vi "Write Config Unitest.vi"(8 "error in (no error)":errorcluster, 11 "main ref":T1) -> (0 "error out":errorcluster)   [LabVIEW 2025]
uses:
  controls/LAB-IQ UI Data.ctl
  Traction Loop/Traction Receipe Enum.ctl
  Config file  FGV Unitest enum.ctl
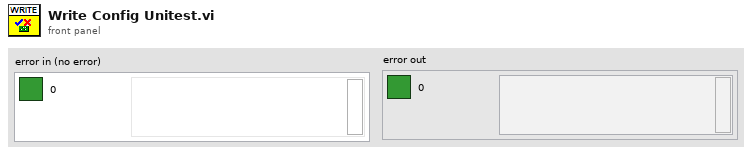
[diagram p1: front panel]
types:
  T1 = typedef "LAB-IQ UI Data.ctl" = cluster{"Main Home Screen":cluster{"GUI":refnum<vi>, "Platform Settings":refnum<vi>, "Configure":refnum<vi>, "Home":refnum<vi>, "EXIT":refnum<vi>, "service 2":refnum<vi>, "MainPage":refnum<vi>, "Analysis":refnum<vi>}, "Platform Settings":cluster{"mm/s  Surge":refnum<vi>, "Update Surge Speed":refnum<vi>, "Drive Error":refnum<vi>, "Disable Axis Jog Soft Limits":refnum<vi>, "mm/s  Sway":refnum<vi>, "Sway and Surge COM Status":refnum<vi>, "Heave COM Status":refnum<vi>, "Enable Platform":refnum<vi>, "Surge Forward Main":refnum<vi>, "Sway Right Main":refnum<vi>, "Sway Left Main":refnum<vi>, "Heave Down Main":refnum<vi>, "Heave Up main":refnum<vi>, "Update Sway Speed":refnum<vi>, "Update Heave Speed":refnum<vi>, "mm/s Heave":refnum<vi>, "mm/sec":refnum<vi>, "mm":refnum<vi>, "Surge Backward Main":refnum<vi>}, "Analysis Screen":cluster{"Analysis Home":refnum<vi>, "Surface Analysis":refnum<vi>, "Imaging":refnum<vi>, "Image Analysis":refnum<vi>, "Post Analysis":refnum<vi>}, "Config Screen":cluster{"Select Load Head":refnum<vi>, "Notes :":refnum<vi>, "FILE":refnum<vi>, "Sample ID :":refnum<vi>, "Operator ID :":refnum<vi>, "Operator Name :":refnum<vi>, "Auto":refnum<vi>}, "Motion Module":cluster{"zNL":refnum<vi>, "NL disp":refnum<vi>, "Rotary Tab":refnum<vi>, "Motion Direction:  3":refnum<vi>, "E.Velocity 2":refnum<vi>, "e.v/ssr 2":refnum<vi>, "Enter Fixed E.Velocity 2":refnum<vi>, "Enter Final SRR 2":refnum<vi>, "Enter initial SRR 2":refnum<vi>, "Enter Fixed SRR 2":refnum<vi>, "Enter the Final E.Velocity (m/s) 2":refnum<vi>, "Enter initial E.Velocity (m/s) 2":refnum<vi>, "Final Speed (RPM) 3":refnum<vi>, "Initial Speed (RPM) 2":refnum<vi>, "Enter the Final Velocity (m/s) 3":refnum<vi>, "Enter initial Velocity (m/s)  3":refnum<vi>, "Ramp Up 2":refnum<vi>, "TEST SELECTION":refnum<vi>, "SPEED SELECTION : ":refnum<vi>, "Angular Oscillation Set":refnum<vi>, "Traction":refnum<vi>, "Step Speed":refnum<vi>, "StepTable For Load-Speed":refnum<vi>, "StepTable For Speed":refnum<vi>, "Surge Forward MM":refnum<vi>, "Surge Backward MM":refnum<vi>, "M3 Image":refnum<vi>, "String 39":refnum<vi>, "Sway Left MM":refnum<vi>, "Sway Right MM":refnum<vi>, "Disable Axis Jog Soft Limits":refnum<vi>, "mm":refnum<vi>, "Heave Down MM":refnum<vi>, "Heave Up MM":refnum<vi>, "Wear Track Diameter (mm)":refnum<vi>, "Set WTD":refnum<vi>, "HomeScratch":refnum<vi>, "HomeRot":refnum<vi>, "PlaceModule":refnum<vi>, "Enter the Angle (Deg)":refnum<vi>, "Enter the Frequency (Hz)":refnum<vi>, "Motion Mode:":refnum<vi>, "LR Sway":refnum<vi>, "Rot Hor":refnum<vi>, "Scratch":refnum<vi>, "LR Cam":refnum<vi>, "MMBack":refnum<vi>, "MMNext":refnum<vi>, "Rot Ver":refnum<vi>, "Rotary Module Selection":refnum<vi>, "calculate rotary":refnum<vi>, "SPEED SELECTION : rotary":refnum<vi>, "Import 2":refnum<vi>, "Save 2":refnum<vi>, "File Path :  2":refnum<vi>, "String 45":refnum<vi>, "StepTable For Speed 3":refnum<vi>, "Enter the Speed(mm/sec)":refnum<vi>, "Enter the Speed(RPM)":refnum<vi>, "Enter Scratch Speed (mm/s):":refnum<vi>, "SwaySpeed Set":refnum<vi>, "Scartch Offset":refnum<vi>, "Motion type:":refnum<vi>, "HomeScratch 2":refnum<vi>, "Enter Scratch length (mm):":refnum<vi>, "Wear Track Diameter":refnum<vi>, "Rotary Speed Exced":refnum<vi>, "Scratch Mode":refnum<vi>, "No of Scratch":refnum<vi>}, "Environmental control":cluster{"Humidity  Status  3":refnum<vi>, "Low Temp  Status  2":refnum<vi>, "TK4 status 2":refnum<vi>, "Stage Temperature":refnum<vi>, "Sample Temperature":refnum<vi>, "Humidity (Amb)":refnum<vi>, "Clear List":refnum<vi>, "Add to list":refnum<vi>, "Wear":refnum<vi>, "Vibration":refnum<vi>, "Humidity (Chamber)":refnum<vi>, "Temperature (Chamber)":refnum<vi>, "ECR ":refnum<vi>, "Temperature (Amb)":refnum<vi>, "Microphone":refnum<vi>, "Acoustic Emission 3":refnum<vi>, "SNext":refnum<vi>, "APBack":refnum<vi>, "Enter the Temperature (°C):":refnum<vi>, "Enter the Stage \nTemperature (°C):":refnum<vi>, "Enter the Humidity (%Rh):":refnum<vi>, "Low Temp":refnum<vi>, "High Temp":refnum<vi>, "Humidity":refnum<vi>, "Sensors Picked":refnum<vi>}, "About Screen":cluster{"Password":refnum<vi>, "Home Service":refnum<vi>, "Advanced Setting":refnum<vi>, "About Tab":refnum<vi>, "ECR Port:":refnum<vi>, "Ramp Port:":refnum<vi>, "Installation/Replacement completed":refnum<vi>, "Loahead":refnum<vi>, "Heave and Surge COM Port:":refnum<vi>, "Sway COM Port:":refnum<vi>, "Temp Modbus:":refnum<vi>, "Humidity Port:":refnum<vi>, "Edit Gain Constants":refnum<vi>, "Save Gain Constants":refnum<vi>}, "Main Screen":cluster{"Main Screen Tab":refnum<vi>, "Angle and Frequency":refnum<vi>, "Stroke (mm)":refnum<vi>, "Angle (Deg)":refnum<vi>, "Main Speed Tab":refnum<vi>, "MTM MOTOR DISPLAY":refnum<vi>, "Disc Speed (m/sec)":refnum<vi>, "Ball Speed (m/sec)":refnum<vi>, "Disc Speed (RPM)":refnum<vi>, "Ball Speed (RPM)":refnum<vi>, "SPEED TAB":refnum<vi>, "Speed (m/sec)":refnum<vi>, "Set Speed (m/sec)":refnum<vi>, "Speed (RPM)":refnum<vi>, "Set Speed":refnum<vi>, "Time Tab":refnum<vi>, "Time ( HH:MM:SS ) 2":refnum<vi>, "Test Duration":refnum<vi>, "Test Duration 4":refnum<vi>, "TEST CYCLE":refnum<vi>, "TOTAL CYCLES":refnum<vi>, "Set Load (N)":refnum<vi>, "Temp Tabs":refnum<vi>, "Heater":refnum<vi>, "TK4 status":refnum<vi>, "ChamberTemp":refnum<vi>, "SetTmp":refnum<vi>, "Controller  Status":refnum<vi>, "ChamberTemp 2":refnum<vi>, "SetTmp 2":refnum<vi>, "Controller  Status 2":refnum<vi>, "ChamberTemp 3":refnum<vi>, "SetTmp 3":refnum<vi>, "Cooling":refnum<vi>, "Load Communication":refnum<vi>, "Ambient \nTemperature":refnum<vi>, "HumCOMStatus":refnum<vi>, "Ambient\n Humidity":refnum<vi>, "Freq (Hz)":refnum<vi>, "Load En":refnum<vi>, "NLt":refnum<vi>, "zNL 2":refnum<vi>, "Humidity On":refnum<vi>, "humidity disp":refnum<vi>, "Set Humidity":refnum<vi>, "NL disp 2":refnum<vi>, "Humidity On 2":refnum<vi>, "humidity disp 2":refnum<vi>, "Set Humidity 2":refnum<vi>, "NL disp 3":refnum<vi>, "AppLoadSeq scratch":refnum<vi>, "Stop Scratch":refnum<vi>, "ClrLog":refnum<vi>, "Trip Log":refnum<vi>, "STOP":refnum<vi>, "Start Test":refnum<vi>, "Test status":refnum<vi>, "AR Led":refnum<vi>, "Data":refnum<vi>, "Health":refnum<vi>, "Sway COM Status":refnum<vi>, "Heave COM Status":refnum<vi>, "Grp Tab":refnum<vi>, "Sub Graph":refnum<vi>, "SD (mm)":refnum<vi>, "Siliding distance Reset Graph":refnum<vi>, "SDGp":refnum<vi>, "Humidity Reset Graph":refnum<vi>, "HumrGp":refnum<vi>, "Acoustic Emission (mV)":refnum<vi>, "Aqucostic Reset Graph":refnum<vi>, "gACQUOS":refnum<vi>, "ECR RESET":refnum<vi>, "ECR":refnum<vi>, "Temperature Reset":refnum<vi>, "Acoustic Emission (mV) 2":refnum<vi>, "Aqucostic Reset Graph 2":refnum<vi>, "gACQUOS 2":refnum<vi>, "ECR RESET 2":refnum<vi>, "ECR 2":refnum<vi>, "Temperature Reset 2":refnum<vi>, "Temperature (deg c)":refnum<vi>, "Speed Reset Graph":refnum<vi>, "Speed Tab":refnum<vi>, "MTM DISC  SPEED":refnum<vi>, "MTM BALL SPEED":refnum<vi>, "speed mm/sec":refnum<vi>, "Hymidity":refnum<vi>, "Humidity Disable trip":refnum<vi>, "CoF Trip  2":refnum<vi>, "Depth Trip":refnum<vi>, "Weart Deapth":refnum<vi>, "Depth Reset Graph":refnum<vi>, "Weart":refnum<vi>, "Depthz":refnum<vi>, "Depth (µm)":refnum<vi>, "WearGp":refnum<vi>, "NL Trip 2":refnum<vi>, "Load pid":refnum<vi>, "Load Disable Trip":refnum<vi>, "Load Reset Graph":refnum<vi>, "NL Display 4":refnum<vi>, "Main Chart 3":refnum<vi>, "BACK":refnum<vi>, "Depth Trip 2":refnum<vi>, "COF TRIP ":refnum<vi>, "Friction Force (N)":refnum<vi>, "FF Reset Graph":refnum<vi>, "FF Disable Trip":refnum<vi>, "FF TRIP":refnum<vi>, "COF Disable Trip":refnum<vi>, "COF Reset Graph":refnum<vi>, "Start Test Temp":refnum<vi>, "zFF":refnum<vi>, "Friction Force (N) Graph":refnum<vi>, "Coefficient of Friction":refnum<vi>, "Scratch Start Test":refnum<vi>, "FF Tab":refnum<vi>, "Cyclic Friction Force (N)":refnum<vi>, "CZ FF":refnum<vi>, "Cyclic Friction Force (N) Graph":refnum<vi>, "Cyclic Coefficient of Friction":refnum<vi>, "Cyclic FF TRIP":refnum<vi>, "Cyclic FF Disable Trip":refnum<vi>, "cyclic COF Disable Trip":refnum<vi>, "cyclic COF TRIP":refnum<vi>, "cyclic COF Reset Graph":refnum<vi>, "Cyclic FF Reset Graph":refnum<vi>, "Test Trip":refnum<vi>, "Multi Scratch Pass":refnum<vi>, "Scratch Start Recording":refnum<vi>}, "Loading":cluster{"Indentation":refnum<vi>, "Reference Sample":refnum<vi>, "Load Cell Communication Slide":refnum<vi>, "com 3":refnum<vi>, "com":refnum<vi>, "DecaForce COM Status":refnum<vi>, "Update":refnum<vi>, "Clear 3":refnum<vi>, "seq":refnum<vi>, "Stribeck table":refnum<vi>, "Stribeck Table  For loading":refnum<vi>, "Loading Mode":refnum<vi>, "Enter the Final Load (N)":refnum<vi>, "Enter the CoF Trip":refnum<vi>, "Enter the Friction Force Trip":refnum<vi>, "Enter the Normal load Trip":refnum<vi>, "Enter the Load  (N)":refnum<vi>, "KiloForce":refnum<vi>, "DecaForce ":refnum<vi>, "MicroForce":refnum<vi>, "LHBack":refnum<vi>, "LHNext":refnum<vi>, "Enter the Loading Rate (N/min)":refnum<vi>, "Message":refnum<vi>, "Warning 2":refnum<vi>, "SSP 0.75":refnum<vi>, "SSP 0.5":refnum<vi>, "SSP 0.3":refnum<vi>, "Warning":refnum<vi>, "gui GIF":refnum<vi>, "Communication is established":refnum<vi>, "AppLoad 4":refnum<vi>, "Multipoint":refnum<vi>, "Load Selection":refnum<vi>}, "PID":cluster{"Ramp MulFac":refnum<vi>, "pulses LoadDiffRamp(2..10)":refnum<vi>, "PulseControlRamp(diff<=3N)":refnum<vi>, "SetLoadDeadband(%) Load(0-10N)":refnum<vi>, "PID gains out delay (microForce)":refnum<vi>, "Ramp":refnum<vi>, "Gain 2":refnum<vi>, "pulses LoadDiff(2..10)":refnum<vi>, "pulses LoadDiff(11..50)":refnum<vi>, "PulseControl(diff<=3N)":refnum<vi>, "SetLoadDeadband(%)  2":refnum<vi>, "Dummy Run":refnum<vi>, "Vertical load (N)":refnum<vi>, "AutoTune":refnum<vi>, "Offset 3 ":refnum<vi>, "apply load":refnum<vi>, "Offset  3":refnum<vi>, "apply load 2":refnum<vi>, "Enter ByPass Load":refnum<vi>, "reinit 3":refnum<vi>, "output range delay":refnum<vi>, "PID gains out delay":refnum<vi>, "Bypass Load":refnum<vi>, "pulsesSent":refnum<vi>, "pulses ":refnum<vi>, "actpid":refnum<vi>, "gFF Rot":refnum<vi>, "pulses LoadDiff(21..1000)":refnum<vi>, "Delay":refnum<vi>, "deadband":refnum<vi>}, "Config Parameters":cluster{"Tab Control 3":refnum<vi>, "Tab Control 19":refnum<vi>, "SAMPLES":refnum<vi>, "Re-initilaize":refnum<vi>, "Filter ON/OFF":refnum<vi>, "TracHomeSurgeOffsetCounts 10MM":refnum<vi>, "TracHomeSwayOffsetCounts 10MM":refnum<vi>, "Acoustic Emission:":refnum<vi>, "Apply Filter (FF)":refnum<vi>, "Filter% 2":refnum<vi>, "Apply Filter (Load)":refnum<vi>, "Filter% ":refnum<vi>, "Sway distance (mm)":refnum<vi>, "Surge distance (mm)":refnum<vi>, "DataSavingLoopDelay(ms)":refnum<vi>, "SAVE 2":refnum<vi>, "Enter Distance":refnum<vi>, "Sway Counts:":refnum<vi>, "Distance (mm): 3":refnum<vi>, "Surge Counts:":refnum<vi>, "Distance (mm): 2":refnum<vi>, "Distance (mm):":refnum<vi>, "Heave Counts:":refnum<vi>, "LRMHomeSurgeOffsetCounts":refnum<vi>, "LRMHomeSwayOffsetCounts":refnum<vi>, "TracHomeSurgeOffsetCounts 20MM":refnum<vi>, "TracHomeSwayOffsetCounts 20MM":refnum<vi>, "RotHomeSwayOffsetCounts":refnum<vi>, "RotHomeSurgeOffsetCounts":refnum<vi>, "Heave distance":refnum<vi>, "Zmm":refnum<vi>, "Heave Pulses/mm":refnum<vi>, "Surge Pulses/mm":refnum<vi>, "Sway Pulses/mm":refnum<vi>, "Heave Pitch":refnum<vi>, "Surge Pitch":refnum<vi>, "Sway Pitch":refnum<vi>, "Heave PPR":refnum<vi>, "Surge PPR":refnum<vi>, "Sway PPR":refnum<vi>, "Tab Control 5":refnum<vi>, "Tab Control 14":refnum<vi>, "Tab Control 26":refnum<vi>, "AE":refnum<vi>, "Heave Loop Delay":refnum<vi>, "Heave PID Speed":refnum<vi>, "Surge Jog Speed":refnum<vi>, "Heave Jog Speed":refnum<vi>, "Sway Loop Delay":refnum<vi>, "Sway PID Speed":refnum<vi>, "Sway Jog Speed":refnum<vi>, "DEPTH TRIP VALUE":refnum<vi>, "LOAD TRIP VALUE":refnum<vi>, "DEPTH TRIP   ENABLE":refnum<vi>, "LOAD TRIP  ENABLE":refnum<vi>, "CYCLIC FF TRIP VALUE":refnum<vi>, "FF TRIP VALUE":refnum<vi>, "CYCLIC CoF TRIP VALUE":refnum<vi>, "COF TRIP VALUE":refnum<vi>, "CYCLIC COF TRIP  ENABLE":refnum<vi>, "CYCLIC FF TRIP  ENABLE":refnum<vi>, "FF TRIP  ENABLE":refnum<vi>, "COF TRIP  ENABLE":refnum<vi>, "JOG TRIP LOAD VALUE (N)":refnum<vi>, "Rotary Vertical":refnum<vi>, "Traction":refnum<vi>, "Scratch":refnum<vi>, "LRM CAM":refnum<vi>, "Sway LRM":refnum<vi>, "Rotary Horizontal":refnum<vi>}, "Loading Com Port":cluster{"ClearAll":refnum<vi>, "Mz(Nm)":refnum<vi>, "My(Nm)":refnum<vi>, "Mx(Nm)":refnum<vi>, "Save Dwell":refnum<vi>, "Mx ":refnum<vi>, "My ":refnum<vi>, "Mz":refnum<vi>, "Fx(N)":refnum<vi>, "Fy(N)":refnum<vi>, "Fz(N)":refnum<vi>, "ZeroAll":refnum<vi>, "Acq Delay (ms)":refnum<vi>, "Burst Delay (ms)":refnum<vi>, "model":refnum<vi>, "SN":refnum<vi>, "FFx(N)":refnum<vi>, "Sensor IP":refnum<vi>, "Port":refnum<vi>, "FFy(N)":refnum<vi>, "Load(N)":refnum<vi>, "delete Handle":refnum<vi>, "Create Handle":refnum<vi>, "ft_data":refnum<vi>, "ft_range":refnum<vi>, "ft_data 2":refnum<vi>, "stop 6":refnum<vi>, "running_flag":refnum<vi>, "ft_udp_handle":refnum<vi>, "get-data-return":refnum<vi>, "get-range-return":refnum<vi>, "zero-return":refnum<vi>, "filter-return":refnum<vi>, "initial-return":refnum<vi>, "deleteHandle-result":refnum<vi>, "Load Cell Temp":refnum<vi>, "Load Cell":refnum<vi>}, "Heave AND Surge":cluster{"SURGE POSE":refnum<vi>, "error out Read":refnum<vi>, "HEAVE POSE":refnum<vi>, "State":refnum<vi>, "Homed":refnum<vi>, "Sequence ID":refnum<vi>, "error out Write":refnum<vi>, "faultCode":refnum<vi>, "Ack ID":refnum<vi>, "SPEED":refnum<vi>, "Distance":refnum<vi>, "Mode Command":refnum<vi>, "Heave and Surge Read":refnum<vi>, "Read Heave Temp":refnum<vi>, "Spare 15":refnum<vi>, "Spare 14":refnum<vi>, "Spare 13":refnum<vi>, "Spare 12":refnum<vi>, "Spare 11":refnum<vi>, "Spare 10":refnum<vi>, "Spare 9":refnum<vi>, "Spare 8":refnum<vi>, "Spare 7":refnum<vi>, "Spare 6":refnum<vi>, "Spare 5":refnum<vi>, "Spare 4":refnum<vi>, "Spare 2":refnum<vi>, "Spare 1":refnum<vi>, "Node Id":refnum<vi>, "Spare 3":refnum<vi>, "SPARE 4":refnum<vi>, "SPARE 3":refnum<vi>, "SPARE 2":refnum<vi>, "SPARE 1":refnum<vi>, "fwMajor":refnum<vi>, "fwMinor":refnum<vi>, "Manual Write":refnum<vi>, "Heave and Surge Write":refnum<vi>, "SPARE 5":refnum<vi>, "Reserved ":refnum<vi>, "SPARE 8":refnum<vi>, "SPARE 6":refnum<vi>, "SPARE 7":refnum<vi>, "SPARE 17":refnum<vi>, "SPARE 16":refnum<vi>, "SPARE 15":refnum<vi>, "SPARE 14":refnum<vi>, "SPARE 13":refnum<vi>, "SPARE 12":refnum<vi>, "SPARE 11":refnum<vi>, "SPARE 10":refnum<vi>, "SPARE 9":refnum<vi>, "System UPTIME":refnum<vi>, "Missed Packets":refnum<vi>, "faultCode Surge Right":refnum<vi>, "faultCode Surge Left":refnum<vi>, "faultCode Heave":refnum<vi>, "UPLINK HEAVE":refnum<vi>, "DOWNLINK HEAVE":refnum<vi>}, "New PID LOGIC":cluster{"Fine Tune Zone":refnum<vi>, "PID SDelay":refnum<vi>, "Max_pos_limit":refnum<vi>, "Min_pos_limit":refnum<vi>, "i_limit":refnum<vi>, "pct_scale":refnum<vi>, "Deadband":refnum<vi>, "Kd":refnum<vi>, "Ki":refnum<vi>, "Kp":refnum<vi>, "Current Position":refnum<vi>, "Set Load":refnum<vi>, "Current Load":refnum<vi>, "Pulse delta":refnum<vi>, "Init Step":refnum<vi>, "Max Step Linit":refnum<vi>, "min_deadband_floor":refnum<vi>, "dynamic_spindle_noise_scalar":refnum<vi>, "min_finetune_floor":refnum<vi>, "filter_alpha":refnum<vi>, "PID":refnum<vi>}, "SWAY ":cluster{"fwMajor":refnum<vi>, "Homed":refnum<vi>, "Rotary POSE":refnum<vi>, "State":refnum<vi>, "SWAY POSE":refnum<vi>, "Ack ID":refnum<vi>, "faultCode":refnum<vi>, "Node Id":refnum<vi>, "fwMinor":refnum<vi>, "Spare 6":refnum<vi>, "Spare 5":refnum<vi>, "Spare 4":refnum<vi>, "Spare 3":refnum<vi>, "Spare 2":refnum<vi>, "Spare 1":refnum<vi>, "Spare 7":refnum<vi>, "SPARE  5":refnum<vi>, "error out Write  SWAY ":refnum<vi>, "error out Read SWAY ":refnum<vi>, "Manual Write SWAY ":refnum<vi>, "SWAY WRITE":refnum<vi>, "SPARE  4":refnum<vi>, "SPARE  3":refnum<vi>, "SPARE 2":refnum<vi>, "SPARE 1":refnum<vi>, "Spare 15":refnum<vi>, "Spare 14":refnum<vi>, "Spare 13":refnum<vi>, "Spare 12":refnum<vi>, "Spare 11":refnum<vi>, "Spare 9":refnum<vi>, "Spare 8":refnum<vi>, "SPEED":refnum<vi>, "Distance":refnum<vi>, "Mode Command":refnum<vi>, "Sequence ID":refnum<vi>, "SWAY READ":refnum<vi>, "Spare 10":refnum<vi>, "Read SWAY Temp":refnum<vi>, "faultCode Sway ":refnum<vi>, "Missed Packets":refnum<vi>, "System UPTIME sway":refnum<vi>, "SPARE 6":refnum<vi>, "SPARE 7":refnum<vi>, "SPARE 9":refnum<vi>, "SPARE 11":refnum<vi>, "SPARE 10":refnum<vi>, "SPARE 8":refnum<vi>, "SPARE 13":refnum<vi>, "SPARE 12":refnum<vi>, "SPARE 17":refnum<vi>, "SPARE 16":refnum<vi>, "SPARE 15":refnum<vi>, "SPARE 14":refnum<vi>, "Reserved":refnum<vi>, "faultCode Rotary":refnum<vi>, "UPLINK SWAY":refnum<vi>, "DOWNLINK SWAY":refnum<vi>}, "Analysis Screen":cluster{"Analysis Home":refnum<vi>, "Refresh 2":refnum<vi>, "MEAN 4":refnum<vi>, "SD 4":refnum<vi>, "VARIANCE 4":refnum<vi>, "MEAN  3":refnum<vi>, "SD  3":refnum<vi>, "VARIANCE  3":refnum<vi>, "MEAN 2":refnum<vi>, "SD  2":refnum<vi>, "VARIANCE 2":refnum<vi>, "MEAN":refnum<vi>, "SD":refnum<vi>, "VARIANCE":refnum<vi>, "File 4 Discription":refnum<vi>, "OPEN 4":refnum<vi>, "File Name 4":refnum<vi>, "OPEN 3":refnum<vi>, "File 3 Discription":refnum<vi>, "File Name 3":refnum<vi>, "Y-AXIS":refnum<vi>, "X-AXIS":refnum<vi>, "XY Graph":refnum<vi>, "File Name 2":refnum<vi>, "File Name 1":refnum<vi>, "OPEN 2":refnum<vi>, "OPEN 1":refnum<vi>, "File 1 Discription ":refnum<vi>, "File 2 Discription":refnum<vi>, "Export":refnum<vi>, "File Format":refnum<vi>}, "Traction":cluster{"faultCode Traction 2":refnum<vi>, "faultCode Traction 1":refnum<vi>, "Missed Packets":refnum<vi>, "System UPTIME Traction":refnum<vi>, "SPARE 17":refnum<vi>, "SPARE 16":refnum<vi>, "SPARE 15":refnum<vi>, "SPARE 14":refnum<vi>, "SPARE 13":refnum<vi>, "SPARE 12":refnum<vi>, "SPARE 11":refnum<vi>, "SPARE 10":refnum<vi>, "SPARE 9":refnum<vi>, "SPARE 8":refnum<vi>, "SPARE 7":refnum<vi>, "SPARE 6":refnum<vi>, "Reserved":refnum<vi>, "SPARE  5":refnum<vi>, "Manual Write TRACTION":refnum<vi>, "TRACTION WRITE":refnum<vi>, "SPARE  4":refnum<vi>, "SPARE  3":refnum<vi>, "SPARE 2":refnum<vi>, "SPARE 1":refnum<vi>, "Spare 7":refnum<vi>, "Spare 6":refnum<vi>, "Spare 5":refnum<vi>, "Spare 4":refnum<vi>, "Spare 2":refnum<vi>, "Spare 1":refnum<vi>, "Node Id":refnum<vi>, "Read TRACTION Temp":refnum<vi>, "fwMinor":refnum<vi>, "fwMajor":refnum<vi>, "faultCode":refnum<vi>, "TRACTION POSE":refnum<vi>, "TRACTION POSE 2":refnum<vi>, "Homed":refnum<vi>, "State":refnum<vi>, "Ack ID":refnum<vi>, "SPEED":refnum<vi>, "Distance":refnum<vi>, "Mode Command":refnum<vi>, "Sequence ID":refnum<vi>, "error out Read TRACTION":refnum<vi>, "error out Write  TRACTION":refnum<vi>, "TRACTION READ":refnum<vi>, "Spare 3":refnum<vi>, "Downlink traction":refnum<vi>, "Uplink Traction":refnum<vi>}, "Traction reciepe":cluster{"SRR Sweep Range (%) Stribeck":refnum<vi>, "Traction Receipe":refnum<vi>, "Total Execution Time":refnum<vi>, "Total Steps":refnum<vi>, "Duration / Step (s)  Stribeck":refnum<vi>, "STRIBECK Fixed SRR List (%)":refnum<vi>, "Duration / Step (s) Traction":refnum<vi>, "SRR Sweep Range (%) traction":refnum<vi>, "Rolling Speed (mm/s)":refnum<vi>, "Temperature Stages (°C)":refnum<vi>, "Ball Load (N)":refnum<vi>, "Lubricant Name":refnum<vi>, "Profile File Name":refnum<vi>, "SET entrainment Velocity":refnum<vi>, "Test Array Size":refnum<vi>, "SRR INDEX [ STRIBECK]":refnum<vi>, "Stribeck Size":refnum<vi>, "SET SRR":refnum<vi>, "ELAPSED TIMER ":refnum<vi>, "BALL SET RPM":refnum<vi>, "DISC SET RPM":refnum<vi>, "SET LOAD":refnum<vi>, "TEMPERATURE READ":refnum<vi>, "SET TEMPERATURE":refnum<vi>, "Traction Size":refnum<vi>, "DISC SPEED (rpm)":refnum<vi>, "BALL SPEED (rpm)":refnum<vi>, "BALL WEAR TRACK":refnum<vi>, "DISC WEARTRACK":refnum<vi>, "SRR INDEX [ TRACTION]":refnum<vi>, "Start Index Type":refnum<vi>, "Enum - Menu":refnum<vi>, "Ball (mm/sec)":refnum<vi>, "Disc (mm/sec)":refnum<vi>}, "Traction Control":cluster{"HomeTraction":refnum<vi>, "Demo Mode Display":refnum<vi>, "Traction Message":refnum<vi>, "Traction Step Update Details":refnum<vi>, "Main Tab sequence for selection":refnum<vi>, "Ramp Tab":refnum<vi>, "e.v/ssr":refnum<vi>, "Enter Fixed E.Velocity":refnum<vi>, "Enter Final SRR":refnum<vi>, "Enter initial SRR":refnum<vi>, "Enter Fixed SRR":refnum<vi>, "Enter the Final E.Velocity (m/s)":refnum<vi>, "Enter initial E.Velocity (m/s)":refnum<vi>, "Ball WTD":refnum<vi>, "E.Velocity":refnum<vi>, "Enter the Final Velocity (m/s)":refnum<vi>, "Enter initial Velocity (m/s)":refnum<vi>, "Ramp Up   Disc":refnum<vi>, "Initial DiscSpeed (RPM)":refnum<vi>, "Final Speed (RPM) Ball":refnum<vi>, "Final Speed (RPM)":refnum<vi>, "Initial Speed (RPM) Ball":refnum<vi>, "Enter the Final Velocity (m/s) Ball":refnum<vi>, "Enter initial Velocity (m/s) Ball":refnum<vi>, "Ramp Up":refnum<vi>, "ExceedBallSpeed step":refnum<vi>, "ExceedDiscSpeed":refnum<vi>, "BallSpeed Exceed Indication":refnum<vi>, "Apply":refnum<vi>, "SPEED SELECTION : MTM":refnum<vi>, "SPEED SELECTION : MTM 2":refnum<vi>, "TEST SELECTION (MTM)":refnum<vi>, "MTM Test Selection":refnum<vi>, "File Path Tab":refnum<vi>, "File Path String":refnum<vi>, "Save":refnum<vi>, "Save  2":refnum<vi>, "Import ":refnum<vi>, "File Path :":refnum<vi>, "Step Sequence Indication Tab":refnum<vi>, "Step Sequence Indication":refnum<vi>, "Calculate Step":refnum<vi>, "StepTable":refnum<vi>, "ExceedDiscSpeed  Cinstant Speed":refnum<vi>, "ExceedBallSpeed Constant":refnum<vi>, "TEST SELECTION (MTM) 2":refnum<vi>, "SPEED SELECTION : MTM 3":refnum<vi>, "MTM Test Selection 2":refnum<vi>, "Enter the Speed (m/sec): ":refnum<vi>, "Enter the Speed (m/sec):  2":refnum<vi>, "Enter the Speed (RPM):":refnum<vi>, "Lower Spped ":refnum<vi>, "Upper":refnum<vi>, "Enter the Speed (RPM):Ball":refnum<vi>, "Disc Motion Direction: ":refnum<vi>, "Ball Motion Direction :":refnum<vi>, "Motion Mode: ":refnum<vi>, "Wear Track Diameter (mm) ":refnum<vi>, "Disc Speed Indicator":refnum<vi>, "ExceedBallSpeed":refnum<vi>}, "Acquostic":cluster{"Last Config Rejected ":refnum<vi>, "rx command count":refnum<vi>, "Current Filter Id":refnum<vi>, "Isolated Gain":refnum<vi>, "DAQ Status":refnum<vi>, "error out":refnum<vi>, "error in (no error)":refnum<vi>, "Uplink Packet":refnum<vi>, "data out":refnum<vi>, "Downlink Packet":refnum<vi>, "Signal Energy":refnum<vi>, "Amplitude db_AE":refnum<vi>, "Peak Amplitude":refnum<vi>, "AE Ring-Down Counts":refnum<vi>, "Gains":refnum<vi>, "Manual Write Acquostic":refnum<vi>}}
  T2 = typedef "Config file  FGV Unitest enum.ctl" = enum16{"OPEN", "READ", "WRITE", "CLOSE"}
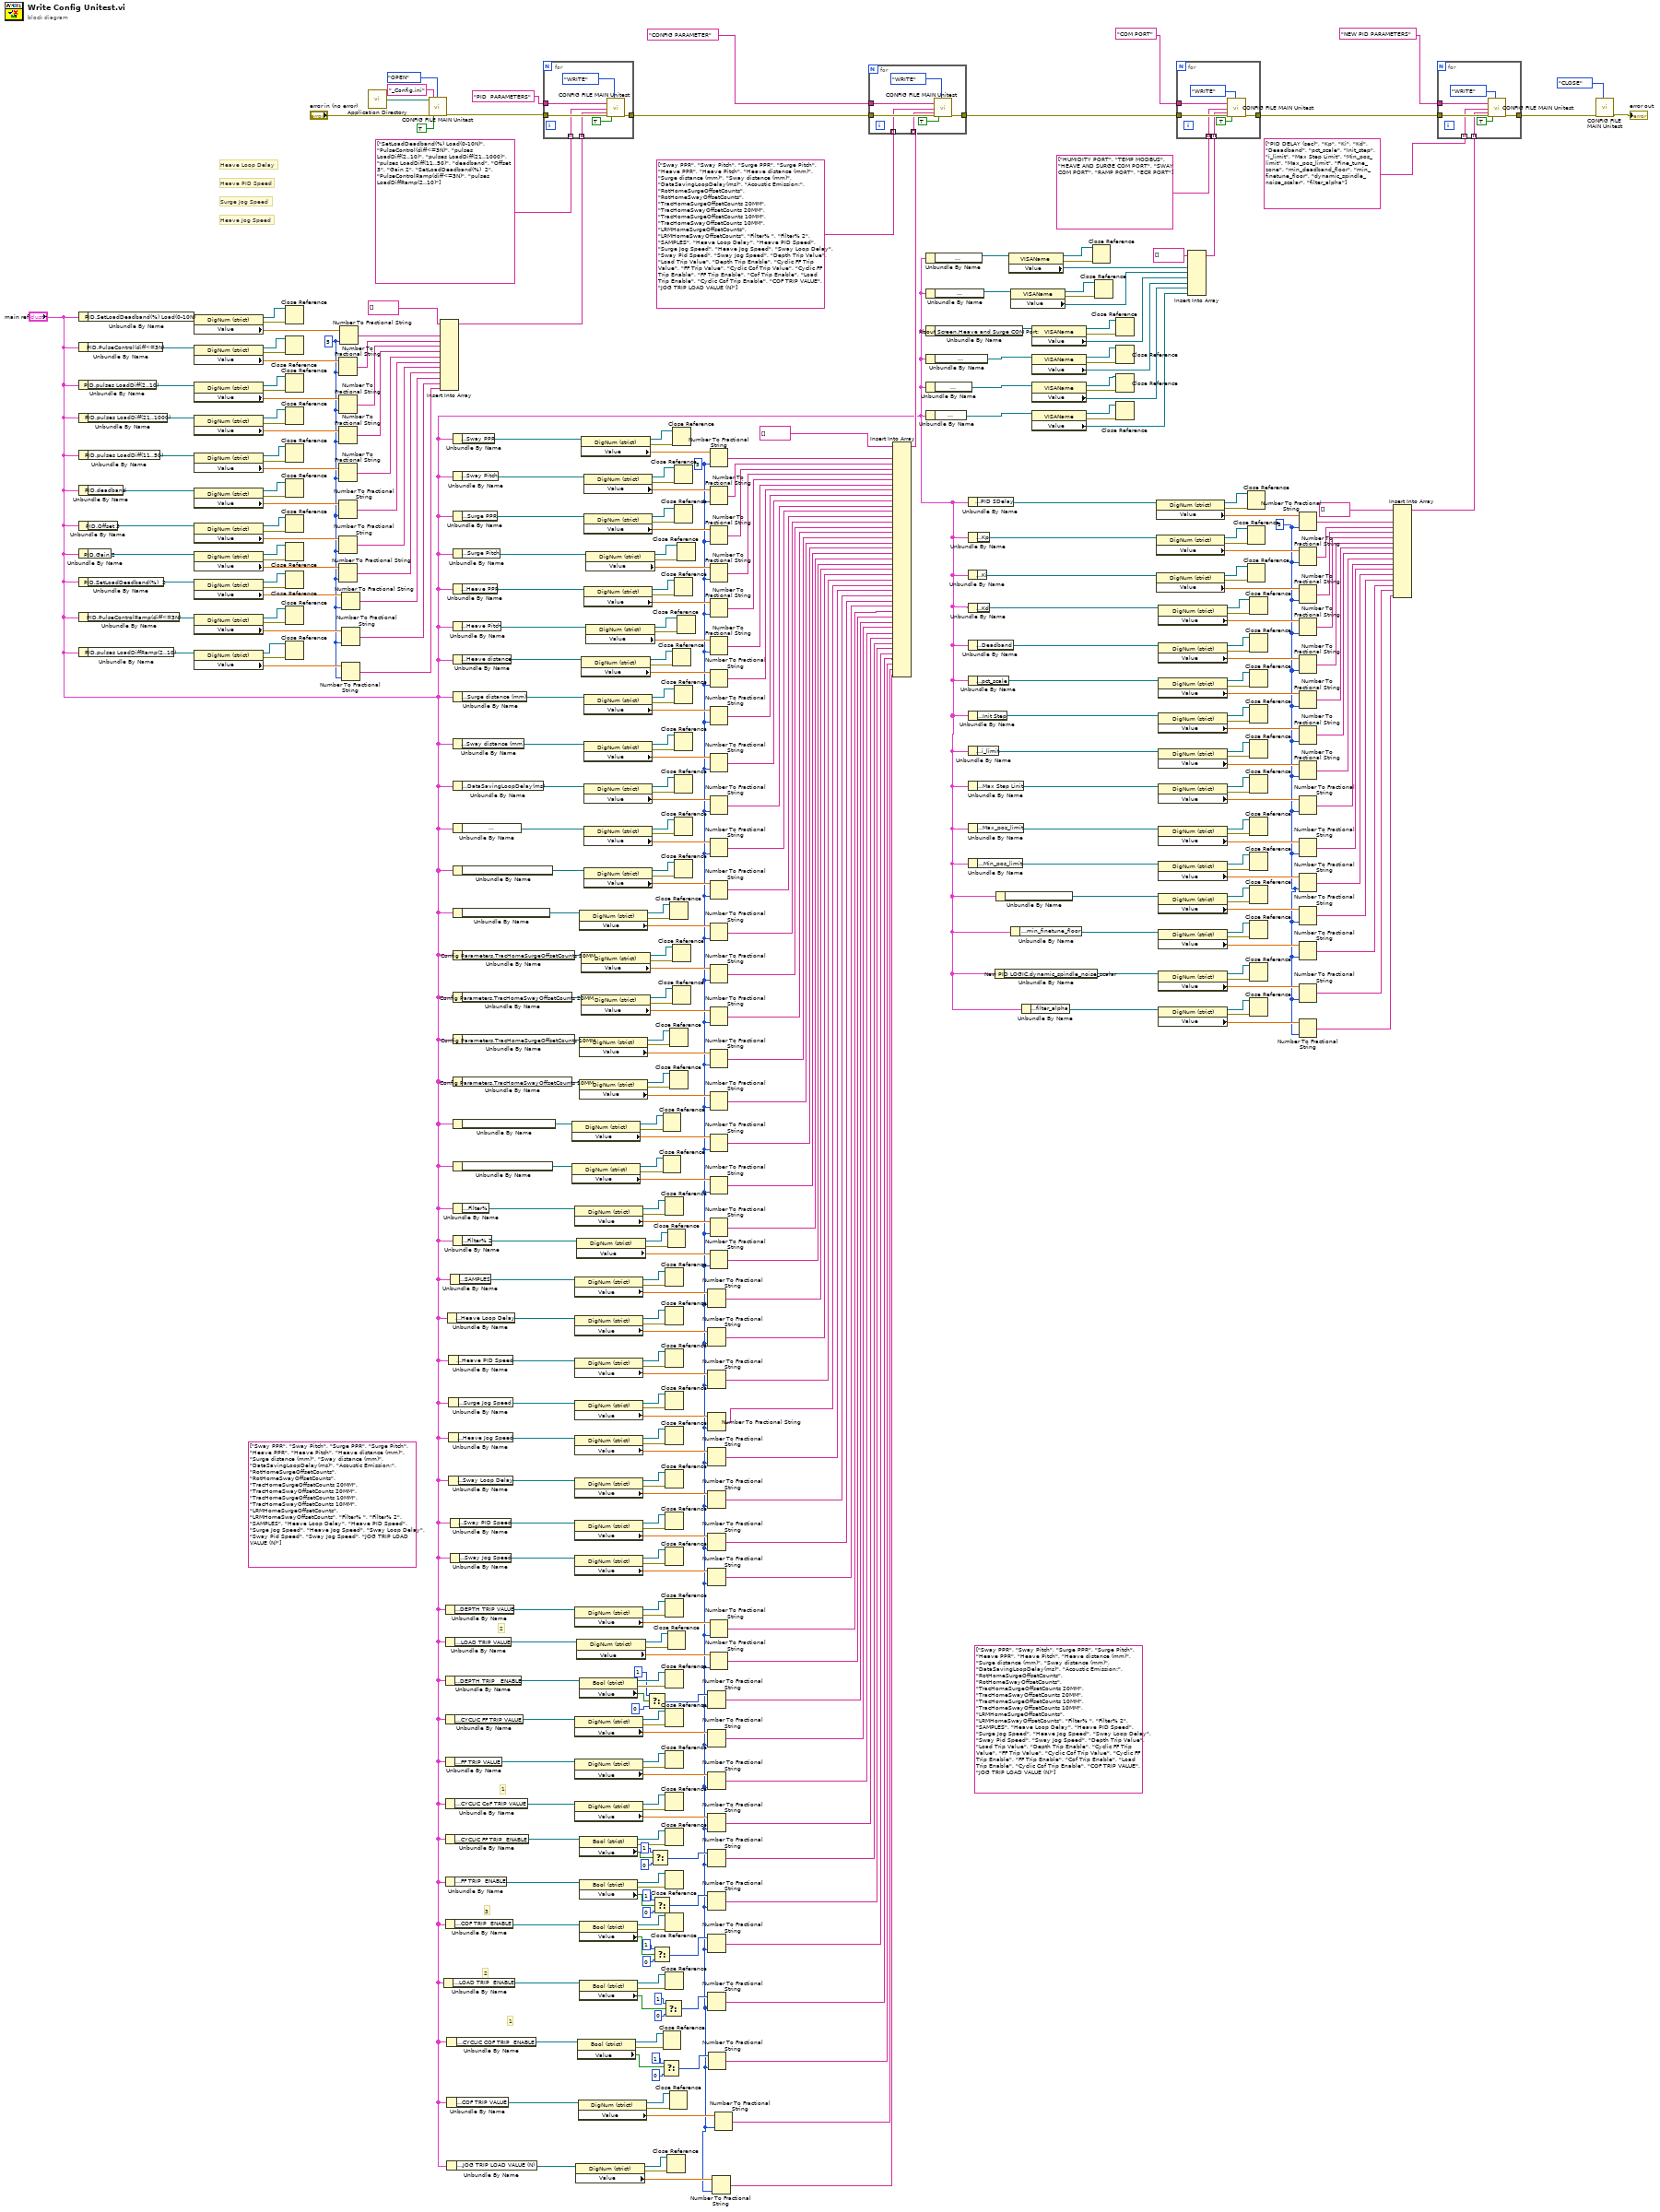
[diagram p0: block diagram]
diagram:
  (unwired) string[] ["Sway PPR", "Sway Pitch", "Surge PPR", "Surge Pitch", "Heave PPR", "Heave Pitch", "Heave distance (mm)", "Surge distance (mm)", "Sway distance (mm)", "DataSavingLoopDelay(ms)", "Acoustic Emission:", "RotHomeSurgeOffsetCounts", "RotHomeSwayOffsetCounts", "TracHomeSurgeOffsetCounts 20MM", "TracHomeSwayOffsetCounts 20MM", "TracHomeSurgeOffsetCounts 10MM", "TracHomeSwayOffsetCounts 10MM", "LRMHomeSurgeOffsetCounts", "LRMHomeSwayOffsetCounts", "Filter% ", "Filter% 2", "SAMPLES", "Heave Loop Delay", "Heave PID Speed", "Surge Jog Speed", "Heave Jog Speed", "Sway Loop Delay", "Sway Pid Speed", "Sway Jog Speed", "JOG TRIP LOAD VALUE (N)"]
  (unwired) string[] ["Sway PPR", "Sway Pitch", "Surge PPR", "Surge Pitch", "Heave PPR", "Heave Pitch", "Heave distance (mm)", "Surge distance (mm)", "Sway distance (mm)", "DataSavingLoopDelay(ms)", "Acoustic Emission:", "RotHomeSurgeOffsetCounts", "RotHomeSwayOffsetCounts", "TracHomeSurgeOffsetCounts 20MM", "TracHomeSwayOffsetCounts 20MM", "TracHomeSurgeOffsetCounts 10MM", "TracHomeSwayOffsetCounts 10MM", "LRMHomeSurgeOffsetCounts", "LRMHomeSwayOffsetCounts", "Filter% ", "Filter% 2", "SAMPLES", "Heave Loop Delay", "Heave PID Speed", "Surge Jog Speed", "Heave Jog Speed", "Sway Loop Delay", "Sway Pid Speed", "Sway Jog Speed", "Depth Trip Value", "Load Trip Value", "Depth Trip Enable", "Cyclic FF Trip Value", "FF Trip Value", "Cyclic Cof Trip Value", "Cyclic FF Trip Enable", "FF Trip Enable", "Cof Trip Enable", "Load Trip Enable", "Cyclic Cof Trip Enable", "COF TRIP VALUE", "JOG TRIP LOAD VALUE (N)"]
  w13 = i16 5 ("precision (6)")
  w3 = i16 5 ("precision (6)")
  w354 = i16 5 ("precision (6)")
  # "3"
  # "2"
  # "2"
  # "1"
  # "1"
  # "Heave Jog Speed"
  # "Surge Jog Speed"
  # "Heave PID Speed"
  # "Heave Loop Delay"
  n1 = Unbundle By Name("main ref") -> ("PID.SetLoadDeadband(%) Load(0-10N)"=w398:refnum<vi>)
  n2 = Unbundle By Name("main ref") -> ("PID.PulseControl(diff<=3N)"=w393:refnum<vi>)
  n3 = Unbundle By Name("main ref") -> ("PID.pulses LoadDiff(2..10)"=w392:refnum<vi>)
  n4 = Unbundle By Name("main ref") -> ("PID.pulses LoadDiff(21..1000)"=w387:refnum<vi>)
  n5 = Unbundle By Name("main ref") -> ("PID.pulses LoadDiff(11..50)"=w386:refnum<vi>)
  n6 = Unbundle By Name("main ref") -> ("PID.deadband"=w381:refnum<vi>)
  n7 = Unbundle By Name("main ref") -> ("PID.Offset 3"=w380:refnum<vi>)
  n8 = Unbundle By Name("main ref") -> ("PID.Gain 2"=w375:refnum<vi>)
  n9 = Unbundle By Name("main ref") -> ("PID.SetLoadDeadband(%)  2"=w374:refnum<vi>)
  n10 = Unbundle By Name("main ref") -> ("PID.PulseControlRamp(diff<=3N)"=w370:refnum<vi>)
  n11 = Unbundle By Name("main ref") -> ("PID.pulses LoadDiffRamp(2..10)"=w368:refnum<vi>)
  n12 = property class="DigNum (strict)"(reference=w398) -> (reference out=w396:refnum<vi>, error out=w397:errorcluster, "Value"=w364:dbl)  [unwired: 1 in]
  n13 = property class="DigNum (strict)"(reference=w393) -> (reference out=w395:refnum<vi>, error out=w394:errorcluster, "Value"=w365:dbl)  [unwired: 1 in]
  n14 = property class="DigNum (strict)"(reference=w392) -> (reference out=w390:refnum<vi>, error out=w391:errorcluster, "Value"=w363:dbl)  [unwired: 1 in]
  n15 = property class="DigNum (strict)"(reference=w387) -> (reference out=w389:refnum<vi>, error out=w388:errorcluster, "Value"=w362:dbl)  [unwired: 1 in]
  n16 = property class="DigNum (strict)"(reference=w386) -> (reference out=w384:refnum<vi>, error out=w385:errorcluster, "Value"=w361:dbl)  [unwired: 1 in]
  n17 = property class="DigNum (strict)"(reference=w381) -> (reference out=w383:refnum<vi>, error out=w382:errorcluster, "Value"=w360:dbl)  [unwired: 1 in]
  n18 = property class="DigNum (strict)"(reference=w380) -> (reference out=w378:refnum<vi>, error out=w379:errorcluster, "Value"=w359:dbl)  [unwired: 1 in]
  n19 = property class="DigNum (strict)"(reference=w375) -> (reference out=w377:refnum<vi>, error out=w376:errorcluster, "Value"=w358:dbl)  [unwired: 1 in]
  n20 = property class="DigNum (strict)"(reference=w374) -> (reference out=w372:refnum<vi>, error out=w373:errorcluster, "Value"=w357:dbl)  [unwired: 1 in]
  n21 = property class="DigNum (strict)"(reference=w370) -> (reference out=w369:refnum<vi>, error out=w371:errorcluster, "Value"=w356:dbl)  [unwired: 1 in]
  n22 = property class="DigNum (strict)"(reference=w368) -> (reference out=w366:refnum<vi>, error out=w367:errorcluster, "Value"=w355:dbl)  [unwired: 1 in]
  n23 = Close Reference(reference=w396, error in (no error)=w397) -> ()  [unwired: 1 out]
  n24 = Close Reference(reference=w395, error in (no error)=w394) -> ()  [unwired: 1 out]
  n25 = Close Reference(reference=w390, error in (no error)=w391) -> ()  [unwired: 1 out]
  n26 = Close Reference(reference=w389, error in (no error)=w388) -> ()  [unwired: 1 out]
  n27 = Close Reference(reference=w384, error in (no error)=w385) -> ()  [unwired: 1 out]
  n28 = Close Reference(reference=w383, error in (no error)=w382) -> ()  [unwired: 1 out]
  n29 = Close Reference(reference=w378, error in (no error)=w379) -> ()  [unwired: 1 out]
  n30 = Close Reference(reference=w377, error in (no error)=w376) -> ()  [unwired: 1 out]
  n31 = Close Reference(reference=w372, error in (no error)=w373) -> ()  [unwired: 1 out]
  n32 = Close Reference(reference=w369, error in (no error)=w371) -> ()  [unwired: 1 out]
  n33 = Close Reference(reference=w366, error in (no error)=w367) -> ()  [unwired: 1 out]
  n34 = Number To Fractional String(number=w365, precision (6)=w354) -> (F-format string=w351:string)  [unwired: 2 in]
  n35 = Number To Fractional String(number=w363, precision (6)=w354) -> (F-format string=w350:string)  [unwired: 2 in]
  n36 = Number To Fractional String(number=w362, precision (6)=w354) -> (F-format string=w349:string)  [unwired: 2 in]
  n37 = Number To Fractional String(number=w361, precision (6)=w354) -> (F-format string=w348:string)  [unwired: 2 in]
  n38 = Number To Fractional String(number=w360, precision (6)=w354) -> (F-format string=w347:string)  [unwired: 2 in]
  n39 = Number To Fractional String(number=w359, precision (6)=w354) -> (F-format string=w346:string)  [unwired: 2 in]
  n40 = Number To Fractional String(number=w358, precision (6)=w354) -> (F-format string=w345:string)  [unwired: 2 in]
  n41 = Number To Fractional String(number=w364, precision (6)=w354) -> (F-format string=w352:string)  [unwired: 2 in]
  n42 = Number To Fractional String(number=w357, precision (6)=w354) -> (F-format string=w344:string)  [unwired: 2 in]
  n43 = Number To Fractional String(number=w356, precision (6)=w354) -> (F-format string=w343:string)  [unwired: 2 in]
  n44 = Number To Fractional String(number=w355, precision (6)=w354) -> (F-format string=w342:string)  [unwired: 2 in]
  n45 = call <vilib>:"Application Directory.vi"() -> ("Application Directory"=w410:path)
  n46 = call "CONFIG FILE MAIN Unitest.vi"("File Path"=w410, "error in"="error in (no error)", "file name"="_Config.ini", "PARAMETER/CONFIG"=TRUE, "Config Enum"=Config_file__FGV_Unitest_enum."OPEN") -> ("error out"=w409:errorcluster)  [unwired: 13 in, 1 out]
  n47 = Insert Into Array(array=string[] [], new element #1=w352, new element #2=w351, new element #3=w350, new element #4=w349, new element #5=w348, new element #6=w347, new element #7=w346, new element #8=w345, new element #9=w344, new element #10=w343, new element #11=w342) -> (w341:string[])  [unwired: 1 in]
  n48 = Unbundle By Name("main ref") -> ("Config Parameters.LOAD TRIP  ENABLE"=w73:refnum<vi>)
  n49 = Unbundle By Name("main ref") -> ("Config Parameters.DEPTH TRIP VALUE"=w77:refnum<vi>)
  n50 = Unbundle By Name("main ref") -> ("Config Parameters.LOAD TRIP VALUE"=w83:refnum<vi>)
  n51 = Unbundle By Name("main ref") -> ("Config Parameters.DEPTH TRIP   ENABLE"=w84:refnum<vi>)
  n52 = Unbundle By Name("main ref") -> ("Config Parameters.CYCLIC FF TRIP VALUE"=w91:refnum<vi>)
  n53 = Unbundle By Name("main ref") -> ("Config Parameters.FF TRIP VALUE"=w92:refnum<vi>)
  n54 = Unbundle By Name("main ref") -> ("Config Parameters.CYCLIC CoF TRIP VALUE"=w99:refnum<vi>)
  n55 = Unbundle By Name("main ref") -> ("Config Parameters.CYCLIC FF TRIP  ENABLE"=w100:refnum<vi>)
  n56 = Unbundle By Name("main ref") -> ("Config Parameters.FF TRIP  ENABLE"=w108:refnum<vi>)
  n57 = Unbundle By Name("main ref") -> ("Config Parameters.COF TRIP  ENABLE"=w103:refnum<vi>)
  n58 = Unbundle By Name("main ref") -> ("Config Parameters.CYCLIC COF TRIP  ENABLE"=w58:refnum<vi>)
  n59 = Unbundle By Name("main ref") -> ("Config Parameters.COF TRIP VALUE"=w36:refnum<vi>)
  n60 = Unbundle By Name("main ref") -> ("Config Parameters.JOG TRIP LOAD VALUE (N)"=w5:refnum<vi>)
  n61 = Unbundle By Name("main ref") -> ("Config Parameters.Heave Loop Delay"=w200:refnum<vi>)
  n62 = Unbundle By Name("main ref") -> ("Config Parameters.Heave PID Speed"=w199:refnum<vi>)
  n63 = Unbundle By Name("main ref") -> ("Config Parameters.Surge Jog Speed"=w192:refnum<vi>)
  n64 = Unbundle By Name("main ref") -> ("Config Parameters.Heave Jog Speed"=w191:refnum<vi>)
  n65 = Unbundle By Name("main ref") -> ("Config Parameters.Sway Loop Delay"=w112:refnum<vi>)
  n66 = Unbundle By Name("main ref") -> ("Config Parameters.SAMPLES"=w258:refnum<vi>)
  n67 = Unbundle By Name("main ref") -> ("Config Parameters.Sway PID Speed"=w119:refnum<vi>)
  n68 = Unbundle By Name("main ref") -> ("Config Parameters.Sway Jog Speed"=w120:refnum<vi>)
  n69 = Unbundle By Name("main ref") -> ("Config Parameters.Sway PPR"=w340:refnum<vi>)
  n70 = Unbundle By Name("main ref") -> ("Config Parameters.Sway Pitch"=w333:refnum<vi>)
  n71 = Unbundle By Name("main ref") -> ("Config Parameters.Surge PPR"=w325:refnum<vi>)
  n72 = Unbundle By Name("main ref") -> ("Config Parameters.Surge Pitch"=w332:refnum<vi>)
  n73 = Unbundle By Name("main ref") -> ("Config Parameters.Heave PPR"=w324:refnum<vi>)
  n74 = Unbundle By Name("main ref") -> ("Config Parameters.Heave Pitch"=w318:refnum<vi>)
  n75 = Unbundle By Name("main ref") -> ("Config Parameters.Heave distance"=w310:refnum<vi>)
  n76 = Unbundle By Name("main ref") -> ("Config Parameters.Surge distance (mm)"=w316:refnum<vi>)
  n77 = Unbundle By Name("main ref") -> ("Config Parameters.Sway distance (mm)"=w307:refnum<vi>)
  n78 = Unbundle By Name("main ref") -> ("Config Parameters.DataSavingLoopDelay(ms)"=w304:refnum<vi>)
  n79 = Unbundle By Name("main ref") -> ("Config Parameters.Acoustic Emission:"=w299:refnum<vi>)
  n80 = Unbundle By Name("main ref") -> ("Config Parameters.RotHomeSurgeOffsetCounts"=w296:refnum<vi>)
  n81 = Unbundle By Name("main ref") -> ("Config Parameters.RotHomeSwayOffsetCounts"=w291:refnum<vi>)
  n82 = Unbundle By Name("main ref") -> ("Config Parameters.TracHomeSurgeOffsetCounts 20MM"=w288:refnum<vi>)
  n83 = Unbundle By Name("main ref") -> ("Config Parameters.TracHomeSwayOffsetCounts 20MM"=w283:refnum<vi>)
  n84 = Unbundle By Name("main ref") -> ("Config Parameters.TracHomeSurgeOffsetCounts 10MM"=w277:refnum<vi>)
  n85 = Unbundle By Name("main ref") -> ("Config Parameters.TracHomeSwayOffsetCounts 10MM"=w282:refnum<vi>)
  n86 = Unbundle By Name("main ref") -> ("Config Parameters.LRMHomeSurgeOffsetCounts"=w271:refnum<vi>)
  n87 = Unbundle By Name("main ref") -> ("Config Parameters.LRMHomeSwayOffsetCounts"=w266:refnum<vi>)
  n88 = Unbundle By Name("main ref") -> ("Config Parameters.Filter%"=w265:refnum<vi>)
  n89 = Unbundle By Name("main ref") -> ("Config Parameters.Filter% 2"=w259:refnum<vi>)
  n90 = for {
    tunnel: w409 -> [w421]
    tunnel: "PID  PARAMETERS" ("WRITE /READ SECTION") -> [w420]
    tunnel: string[] ["SetLoadDeadband(%) Load(0-10N)", "PulseControl(diff<=3N)", "pulses LoadDiff(2..10)", "pulses LoadDiff(21..1000)", "pulses LoadDiff(11..50)", "deadband", "Offset  3", "Gain 2", "SetLoadDeadband(%)  2", "PulseControlRamp(diff<=3N)", "pulses LoadDiffRamp(2..10)"] -> [w417] mode=indexing
    tunnel: [w419] -> w406
    tunnel: w341 -> [w416] mode=indexing
    n91 = call "CONFIG FILE MAIN Unitest.vi"("WRITE /READ SECTION"=w420, "WRITE KEY"=w417, "WRITE VALUE"=w416, "error in"=w421, "PARAMETER/CONFIG"=TRUE, "Config Enum"=Config_file__FGV_Unitest_enum."WRITE") -> ("error out"=w419:errorcluster)  [unwired: 12 in, 1 out]
  }
  n92 = property class="DigNum (strict)"(reference=w271) -> (reference out=w272:refnum<vi>, error out=w270:errorcluster, "Value"=w269:dbl)  [unwired: 1 in]
  n93 = property class="DigNum (strict)"(reference=w266) -> (reference out=w273:refnum<vi>, error out=w267:errorcluster, "Value"=w268:dbl)  [unwired: 1 in]
  n94 = property class="DigNum (strict)"(reference=w265) -> (reference out=w262:refnum<vi>, error out=w264:errorcluster, "Value"=w263:dbl)  [unwired: 1 in]
  n95 = property class="DigNum (strict)"(reference=w258) -> (reference out=w255:refnum<vi>, error out=w257:errorcluster, "Value"=w256:dbl)  [unwired: 1 in]
  n96 = property class="DigNum (strict)"(reference=w200) -> (reference out=w203:refnum<vi>, error out=w201:errorcluster, "Value"=w202:dbl)  [unwired: 1 in]
  n97 = property class="DigNum (strict)"(reference=w199) -> (reference out=w196:refnum<vi>, error out=w198:errorcluster, "Value"=w197:dbl)  [unwired: 1 in]
  n98 = property class="DigNum (strict)"(reference=w192) -> (reference out=w195:refnum<vi>, error out=w193:errorcluster, "Value"=w194:dbl)  [unwired: 1 in]
  n99 = property class="DigNum (strict)"(reference=w191) -> (reference out=w188:refnum<vi>, error out=w190:errorcluster, "Value"=w189:dbl)  [unwired: 1 in]
  n100 = property class="DigNum (strict)"(reference=w112) -> (reference out=w115:refnum<vi>, error out=w113:errorcluster, "Value"=w114:dbl)  [unwired: 1 in]
  n101 = property class="DigNum (strict)"(reference=w119) -> (reference out=w116:refnum<vi>, error out=w118:errorcluster, "Value"=w117:dbl)  [unwired: 1 in]
  n102 = property class="DigNum (strict)"(reference=w120) -> (reference out=w123:refnum<vi>, error out=w121:errorcluster, "Value"=w122:dbl)  [unwired: 1 in]
  n103 = property class="DigNum (strict)"(reference=w77) -> (reference out=w80:refnum<vi>, error out=w78:errorcluster, "Value"=w79:dbl)  [unwired: 1 in]
  n104 = property class="DigNum (strict)"(reference=w91) -> (reference out=w88:refnum<vi>, error out=w90:errorcluster, "Value"=w89:dbl)  [unwired: 1 in]
  n105 = property class="DigNum (strict)"(reference=w92) -> (reference out=w95:refnum<vi>, error out=w93:errorcluster, "Value"=w94:dbl)  [unwired: 1 in]
  n106 = property class="DigNum (strict)"(reference=w99) -> (reference out=w96:refnum<vi>, error out=w98:errorcluster, "Value"=w97:dbl)  [unwired: 1 in]
  n107 = property class="DigNum (strict)"(reference=w5) -> (reference out=w7:refnum<vi>, error out=w6:errorcluster, "Value"=w8:dbl)  [unwired: 1 in]
  n108 = property class="DigNum (strict)"(reference=w259) -> (reference out=w254:refnum<vi>, error out=w260:errorcluster, "Value"=w261:dbl)  [unwired: 1 in]
  n109 = property class="DigNum (strict)"(reference=w83) -> (reference out=w87:refnum<vi>, error out=w82:errorcluster, "Value"=w81:dbl)  [unwired: 1 in]
  n110 = property class="Bool (strict)"(reference=w58) -> (reference out=w60:refnum<vi>, error out=w59:errorcluster, "Value"=w49:bool)  [unwired: 1 in]
  n111 = property class="DigNum (strict)"(reference=w36) -> (reference out=w34:refnum<vi>, error out=w35:errorcluster, "Value"=w33:dbl)  [unwired: 1 in]
  n112 = property class="DigNum (strict)"(reference=w291) -> (reference out=w290:refnum<vi>, error out=w292:errorcluster, "Value"=w293:dbl)  [unwired: 1 in]
  n113 = property class="DigNum (strict)"(reference=w277) -> (reference out=w275:refnum<vi>, error out=w278:errorcluster, "Value"=w279:dbl)  [unwired: 1 in]
  n114 = property class="DigNum (strict)"(reference=w282) -> (reference out=w274:refnum<vi>, error out=w281:errorcluster, "Value"=w280:dbl)  [unwired: 1 in]
  n115 = property class="Bool (strict)"(reference=w84) -> (reference out=w86:refnum<vi>, error out=w85:errorcluster, "Value"=w76:bool)  [unwired: 1 in]
  n116 = property class="Bool (strict)"(reference=w100) -> (reference out=w102:refnum<vi>, error out=w101:errorcluster, "Value"=w54:bool)  [unwired: 1 in]
  n117 = property class="Bool (strict)"(reference=w108) -> (reference out=w106:refnum<vi>, error out=w107:errorcluster, "Value"=w55:bool)  [unwired: 1 in]
  n118 = property class="Bool (strict)"(reference=w103) -> (reference out=w105:refnum<vi>, error out=w104:errorcluster, "Value"=w56:bool)  [unwired: 1 in]
  n119 = property class="Bool (strict)"(reference=w73) -> (reference out=w71:refnum<vi>, error out=w72:errorcluster, "Value"=w57:bool)  [unwired: 1 in]
  n120 = property class="DigNum (strict)"(reference=w340) -> (reference out=w338:refnum<vi>, error out=w339:errorcluster, "Value"=w337:dbl)  [unwired: 1 in]
  n121 = property class="DigNum (strict)"(reference=w310) -> (reference out=w229:refnum<vi>, error out=w311:errorcluster, "Value"=w312:dbl)  [unwired: 1 in]
  n122 = property class="DigNum (strict)"(reference=w288) -> (reference out=w289:refnum<vi>, error out=w287:errorcluster, "Value"=w286:dbl)  [unwired: 1 in]
  n123 = property class="DigNum (strict)"(reference=w283) -> (reference out=w276:refnum<vi>, error out=w284:errorcluster, "Value"=w285:dbl)  [unwired: 1 in]
  n124 = property class="DigNum (strict)"(reference=w333) -> (reference out=w335:refnum<vi>, error out=w334:errorcluster, "Value"=w336:dbl)  [unwired: 1 in]
  n125 = property class="DigNum (strict)"(reference=w325) -> (reference out=w327:refnum<vi>, error out=w326:errorcluster, "Value"=w328:dbl)  [unwired: 1 in]
  n126 = property class="DigNum (strict)"(reference=w324) -> (reference out=w317:refnum<vi>, error out=w323:errorcluster, "Value"=w322:dbl)  [unwired: 1 in]
  n127 = property class="DigNum (strict)"(reference=w316) -> (reference out=w314:refnum<vi>, error out=w315:errorcluster, "Value"=w313:dbl)  [unwired: 1 in]
  n128 = property class="DigNum (strict)"(reference=w307) -> (reference out=w306:refnum<vi>, error out=w308:errorcluster, "Value"=w309:dbl)  [unwired: 1 in]
  n129 = property class="DigNum (strict)"(reference=w304) -> (reference out=w305:refnum<vi>, error out=w303:errorcluster, "Value"=w302:dbl)  [unwired: 1 in]
  n130 = property class="DigNum (strict)"(reference=w299) -> (reference out=w298:refnum<vi>, error out=w300:errorcluster, "Value"=w301:dbl)  [unwired: 1 in]
  n131 = property class="DigNum (strict)"(reference=w296) -> (reference out=w297:refnum<vi>, error out=w295:errorcluster, "Value"=w294:dbl)  [unwired: 1 in]
  n132 = property class="DigNum (strict)"(reference=w332) -> (reference out=w330:refnum<vi>, error out=w331:errorcluster, "Value"=w329:dbl)  [unwired: 1 in]
  n133 = property class="DigNum (strict)"(reference=w318) -> (reference out=w320:refnum<vi>, error out=w319:errorcluster, "Value"=w321:dbl)  [unwired: 1 in]
  n134 = Select(t=1, s=w76, f=0) -> (s? t:f=w31:i32)
  n135 = Select(t=1, s=w54, f=0) -> (s? t:f=w53:i32)
  n136 = Select(t=1, s=w55, f=0) -> (s? t:f=w52:i32)
  n137 = Select(t=1, s=w56, f=0) -> (s? t:f=w51:i32)
  n138 = Select(t=1, s=w49, f=0) -> (s? t:f=w48:i32)
  n139 = Close Reference(reference=w272, error in (no error)=w270) -> ()  [unwired: 1 out]
  n140 = Close Reference(reference=w273, error in (no error)=w267) -> ()  [unwired: 1 out]
  n141 = Close Reference(reference=w60, error in (no error)=w59) -> ()  [unwired: 1 out]
  n142 = Select(t=1, s=w57, f=0) -> (s? t:f=w50:i32)
  n143 = Close Reference(reference=w262, error in (no error)=w264) -> ()  [unwired: 1 out]
  n144 = Close Reference(reference=w255, error in (no error)=w257) -> ()  [unwired: 1 out]
  n145 = Close Reference(reference=w203, error in (no error)=w201) -> ()  [unwired: 1 out]
  n146 = Close Reference(reference=w196, error in (no error)=w198) -> ()  [unwired: 1 out]
  n147 = Close Reference(reference=w195, error in (no error)=w193) -> ()  [unwired: 1 out]
  n148 = Close Reference(reference=w188, error in (no error)=w190) -> ()  [unwired: 1 out]
  n149 = Close Reference(reference=w115, error in (no error)=w113) -> ()  [unwired: 1 out]
  n150 = Close Reference(reference=w116, error in (no error)=w118) -> ()  [unwired: 1 out]
  n151 = Close Reference(reference=w123, error in (no error)=w121) -> ()  [unwired: 1 out]
  n152 = Close Reference(reference=w80, error in (no error)=w78) -> ()  [unwired: 1 out]
  n153 = Close Reference(reference=w86, error in (no error)=w85) -> ()  [unwired: 1 out]
  n154 = Close Reference(reference=w88, error in (no error)=w90) -> ()  [unwired: 1 out]
  n155 = Close Reference(reference=w95, error in (no error)=w93) -> ()  [unwired: 1 out]
  n156 = Close Reference(reference=w96, error in (no error)=w98) -> ()  [unwired: 1 out]
  n157 = Close Reference(reference=w102, error in (no error)=w101) -> ()  [unwired: 1 out]
  n158 = Close Reference(reference=w106, error in (no error)=w107) -> ()  [unwired: 1 out]
  n159 = Close Reference(reference=w105, error in (no error)=w104) -> ()  [unwired: 1 out]
  n160 = Close Reference(reference=w71, error in (no error)=w72) -> ()  [unwired: 1 out]
  n161 = Close Reference(reference=w7, error in (no error)=w6) -> ()  [unwired: 1 out]
  n162 = Close Reference(reference=w254, error in (no error)=w260) -> ()  [unwired: 1 out]
  n163 = Close Reference(reference=w87, error in (no error)=w82) -> ()  [unwired: 1 out]
  n164 = Close Reference(reference=w34, error in (no error)=w35) -> ()  [unwired: 1 out]
  n165 = Close Reference(reference=w290, error in (no error)=w292) -> ()  [unwired: 1 out]
  n166 = Close Reference(reference=w275, error in (no error)=w278) -> ()  [unwired: 1 out]
  n167 = Close Reference(reference=w274, error in (no error)=w281) -> ()  [unwired: 1 out]
  n168 = Close Reference(reference=w338, error in (no error)=w339) -> ()  [unwired: 1 out]
  n169 = Close Reference(reference=w229, error in (no error)=w311) -> ()  [unwired: 1 out]
  n170 = Close Reference(reference=w289, error in (no error)=w287) -> ()  [unwired: 1 out]
  n171 = Close Reference(reference=w276, error in (no error)=w284) -> ()  [unwired: 1 out]
  n172 = Close Reference(reference=w335, error in (no error)=w334) -> ()  [unwired: 1 out]
  n173 = Close Reference(reference=w327, error in (no error)=w326) -> ()  [unwired: 1 out]
  n174 = Close Reference(reference=w317, error in (no error)=w323) -> ()  [unwired: 1 out]
  n175 = Close Reference(reference=w314, error in (no error)=w315) -> ()  [unwired: 1 out]
  n176 = Close Reference(reference=w306, error in (no error)=w308) -> ()  [unwired: 1 out]
  n177 = Close Reference(reference=w305, error in (no error)=w303) -> ()  [unwired: 1 out]
  n178 = Close Reference(reference=w298, error in (no error)=w300) -> ()  [unwired: 1 out]
  n179 = Close Reference(reference=w297, error in (no error)=w295) -> ()  [unwired: 1 out]
  n180 = Close Reference(reference=w330, error in (no error)=w331) -> ()  [unwired: 1 out]
  n181 = Close Reference(reference=w320, error in (no error)=w319) -> ()  [unwired: 1 out]
  n182 = Number To Fractional String(number=w256, precision (6)=w3) -> (F-format string=w231:string)  [unwired: 2 in]
  n183 = Number To Fractional String(number=w202, precision (6)=w3) -> (F-format string=w187:string)  [unwired: 2 in]
  n184 = Number To Fractional String(number=w197, precision (6)=w3) -> (F-format string=w186:string)  [unwired: 2 in]
  n185 = Number To Fractional String(number=w194, precision (6)=w3) -> (F-format string=w185:string)  [unwired: 2 in]
  n186 = Number To Fractional String(number=w189, precision (6)=w3) -> (F-format string=w184:string)  [unwired: 2 in]
  n187 = Number To Fractional String(number=w114, precision (6)=w3) -> (F-format string=w111:string)  [unwired: 2 in]
  n188 = Number To Fractional String(number=w117, precision (6)=w3) -> (F-format string=w110:string)  [unwired: 2 in]
  n189 = Number To Fractional String(number=w122, precision (6)=w3) -> (F-format string=w109:string)  [unwired: 2 in]
  n190 = Number To Fractional String(number=w31, precision (6)=w3) -> (F-format string=w45:string)  [unwired: 2 in]
  n191 = Number To Fractional String(number=w89, precision (6)=w3) -> (F-format string=w44:string)  [unwired: 2 in]
  n192 = Number To Fractional String(number=w94, precision (6)=w3) -> (F-format string=w43:string)  [unwired: 2 in]
  n193 = Number To Fractional String(number=w97, precision (6)=w3) -> (F-format string=w42:string)  [unwired: 2 in]
  n194 = Number To Fractional String(number=w53, precision (6)=w3) -> (F-format string=w41:string)  [unwired: 2 in]
  n195 = Number To Fractional String(number=w52, precision (6)=w3) -> (F-format string=w40:string)  [unwired: 2 in]
  n196 = Number To Fractional String(number=w51, precision (6)=w3) -> (F-format string=w39:string)  [unwired: 2 in]
  n197 = Number To Fractional String(number=w50, precision (6)=w3) -> (F-format string=w38:string)  [unwired: 2 in]
  n198 = Number To Fractional String(number=w48, precision (6)=w3) -> (F-format string=w37:string)  [unwired: 2 in]
  n199 = Number To Fractional String(number=w337, precision (6)=w3) -> (F-format string=w252:string)  [unwired: 2 in]
  n200 = Number To Fractional String(number=w336, precision (6)=w3) -> (F-format string=w251:string)  [unwired: 2 in]
  n201 = Number To Fractional String(number=w328, precision (6)=w3) -> (F-format string=w250:string)  [unwired: 2 in]
  n202 = Number To Fractional String(number=w329, precision (6)=w3) -> (F-format string=w249:string)  [unwired: 2 in]
  n203 = Number To Fractional String(number=w322, precision (6)=w3) -> (F-format string=w248:string)  [unwired: 2 in]
  n204 = Number To Fractional String(number=w321, precision (6)=w3) -> (F-format string=w247:string)  [unwired: 2 in]
  n205 = Number To Fractional String(number=w312, precision (6)=w3) -> (F-format string=w246:string)  [unwired: 2 in]
  n206 = Number To Fractional String(number=w313, precision (6)=w3) -> (F-format string=w245:string)  [unwired: 2 in]
  n207 = Number To Fractional String(number=w309, precision (6)=w3) -> (F-format string=w244:string)  [unwired: 2 in]
  n208 = Number To Fractional String(number=w302, precision (6)=w3) -> (F-format string=w243:string)  [unwired: 2 in]
  n209 = Number To Fractional String(number=w301, precision (6)=w3) -> (F-format string=w242:string)  [unwired: 2 in]
  n210 = Number To Fractional String(number=w294, precision (6)=w3) -> (F-format string=w241:string)  [unwired: 2 in]
  n211 = Number To Fractional String(number=w293, precision (6)=w3) -> (F-format string=w240:string)  [unwired: 2 in]
  n212 = Number To Fractional String(number=w286, precision (6)=w3) -> (F-format string=w239:string)  [unwired: 2 in]
  n213 = Number To Fractional String(number=w285, precision (6)=w3) -> (F-format string=w238:string)  [unwired: 2 in]
  n214 = Number To Fractional String(number=w279, precision (6)=w3) -> (F-format string=w237:string)  [unwired: 2 in]
  n215 = Number To Fractional String(number=w280, precision (6)=w3) -> (F-format string=w236:string)  [unwired: 2 in]
  n216 = Number To Fractional String(number=w269, precision (6)=w3) -> (F-format string=w235:string)  [unwired: 2 in]
  n217 = Number To Fractional String(number=w268, precision (6)=w3) -> (F-format string=w234:string)  [unwired: 2 in]
  n218 = Number To Fractional String(number=w263, precision (6)=w3) -> (F-format string=w233:string)  [unwired: 2 in]
  n219 = Number To Fractional String(number=w261, precision (6)=w3) -> (F-format string=w232:string)  [unwired: 2 in]
  n220 = Number To Fractional String(number=w79, precision (6)=w3) -> (F-format string=w47:string)  [unwired: 2 in]
  n221 = Number To Fractional String(number=w81, precision (6)=w3) -> (F-format string=w46:string)  [unwired: 2 in]
  n222 = Number To Fractional String(number=w8, precision (6)=w3) -> (F-format string=w2:string)  [unwired: 2 in]
  n223 = Number To Fractional String(number=w33, precision (6)=w3) -> (F-format string=w32:string)  [unwired: 2 in]
  n224 = Insert Into Array(array=string[] [], new element #1=w252, new element #2=w251, new element #3=w250, new element #4=w249, new element #5=w248, new element #6=w247, new element #7=w246, new element #8=w245, new element #9=w244, new element #10=w243, new element #11=w242, new element #12=w241, new element #13=w240, new element #14=w239, new element #15=w238, new element #16=w237, new element #17=w236, new element #18=w235, new element #19=w234, new element #20=w233, new element #21=w232, new element #22=w231, new element #23=w187, new element #24=w186, new element #25=w185, new element #26=w184, new element #27=w111, new element #28=w110, new element #29=w109, new element #30=w47, new element #31=w46, new element #32=w45, new element #33=w44, new element #34=w43, new element #35=w42, new element #36=w41, new element #37=w40, new element #38=w39, new element #39=w38, new element #40=w37, new element #41=w32, new element #42=w2) -> (w230:string[])  [unwired: 1 in]
  n225 = for {
    tunnel: w406 -> [w428]
    tunnel: "CONFIG PARAMETER" ("WRITE /READ SECTION") -> [w427]
    tunnel: [w426] -> w404
    tunnel: string[] ["Sway PPR", "Sway Pitch", "Surge PPR", "Surge Pitch", "Heave PPR", "Heave Pitch", "Heave distance (mm)", "Surge distance (mm)", "Sway distance (mm)", "DataSavingLoopDelay(ms)", "Acoustic Emission:", "RotHomeSurgeOffsetCounts", "RotHomeSwayOffsetCounts", "TracHomeSurgeOffsetCounts 20MM", "TracHomeSwayOffsetCounts 20MM", "TracHomeSurgeOffsetCounts 10MM", "TracHomeSwayOffsetCounts 10MM", "LRMHomeSurgeOffsetCounts", "LRMHomeSwayOffsetCounts", "Filter% ", "Filter% 2", "SAMPLES", "Heave Loop Delay", "Heave PID Speed", "Surge Jog Speed", "Heave Jog Speed", "Sway Loop Delay", "Sway Pid Speed", "Sway Jog Speed", "Depth Trip Value", "Load Trip Value", "Depth Trip Enable", "Cyclic FF Trip Value", "FF Trip Value", "Cyclic Cof Trip Value", "Cyclic FF Trip Enable", "FF Trip Enable", "Cof Trip Enable", "Load Trip Enable", "Cyclic Cof Trip Enable", "COF TRIP VALUE", "JOG TRIP LOAD VALUE (N)"] -> [w424] mode=indexing
    tunnel: w230 -> [w422] mode=indexing
    n226 = call "CONFIG FILE MAIN Unitest.vi"("WRITE /READ SECTION"=w427, "WRITE KEY"=w424, "WRITE VALUE"=w422, "error in"=w428, "PARAMETER/CONFIG"=TRUE, "Config Enum"=Config_file__FGV_Unitest_enum."WRITE") -> ("error out"=w426:errorcluster)  [unwired: 12 in, 1 out]
  }
  n227 = Unbundle By Name("main ref") -> ("About Screen.Humidity Port:"=w227:refnum<vi>)
  n228 = Unbundle By Name("main ref") -> ("About Screen.Temp Modbus:"=w222:refnum<vi>)
  n229 = Unbundle By Name("main ref") -> ("About Screen.Heave and Surge COM Port:"=w219:refnum<vi>)
  n230 = Unbundle By Name("main ref") -> ("About Screen.Sway COM Port:"=w215:refnum<vi>)
  n231 = Unbundle By Name("main ref") -> ("About Screen.Ramp Port:"=w214:refnum<vi>)
  n232 = Unbundle By Name("main ref") -> ("About Screen.ECR Port:"=w211:refnum<vi>)
  n233 = Unbundle By Name("main ref") -> ("New PID LOGIC.PID SDelay"=w178:refnum<vi>)
  n234 = Unbundle By Name("main ref") -> ("New PID LOGIC.Kp"=w177:refnum<vi>)
  n235 = Unbundle By Name("main ref") -> ("New PID LOGIC.Ki"=w172:refnum<vi>)
  n236 = Unbundle By Name("main ref") -> ("New PID LOGIC.Kd"=w171:refnum<vi>)
  n237 = Unbundle By Name("main ref") -> ("New PID LOGIC.Deadband"=w167:refnum<vi>)
  n238 = Unbundle By Name("main ref") -> ("New PID LOGIC.pct_scale"=w166:refnum<vi>)
  n239 = Unbundle By Name("main ref") -> ("New PID LOGIC.Init Step"=w163:refnum<vi>)
  n240 = Unbundle By Name("main ref") -> ("New PID LOGIC.i_limit"=w162:refnum<vi>)
  n241 = Unbundle By Name("main ref") -> ("New PID LOGIC.Max Step Linit"=w159:refnum<vi>)
  n242 = Unbundle By Name("main ref") -> ("New PID LOGIC.Max_pos_limit"=w157:refnum<vi>)
  n243 = Unbundle By Name("main ref") -> ("New PID LOGIC.Min_pos_limit"=w156:refnum<vi>)
  n244 = Unbundle By Name("main ref") -> ("New PID LOGIC.dynamic_spindle_noise_scalar"=w19:refnum<vi>)
  n245 = Unbundle By Name("main ref") -> ("New PID LOGIC.min_deadband_floor"=w14:refnum<vi>)
  n246 = property class="VISAName"(reference=w227) -> (reference out=w225:refnum<vi>, error out=w226:errorcluster, "Value"=w221:refnum<visa-resource-name>)  [unwired: 1 in]
  n247 = property class="VISAName"(reference=w222) -> (reference out=w224:refnum<vi>, error out=w223:errorcluster, "Value"=w220:refnum<visa-resource-name>)  [unwired: 1 in]
  n248 = Unbundle By Name("main ref") -> ("New PID LOGIC.min_finetune_floor"=w17:refnum<vi>)
  n249 = Unbundle By Name("main ref") -> ("New PID LOGIC.filter_alpha"=w20:refnum<vi>)
  n250 = property class="VISAName"(reference=w219) -> (reference out=w217:refnum<vi>, error out=w218:errorcluster, "Value"=w210:refnum<visa-resource-name>)  [unwired: 1 in]
  n251 = property class="VISAName"(reference=w215) -> (reference out=w209:refnum<vi>, error out=w216:errorcluster, "Value"=w208:refnum<visa-resource-name>)  [unwired: 1 in]
  n252 = property class="VISAName"(reference=w214) -> (reference out=w205:refnum<vi>, error out=w213:errorcluster, "Value"=w207:refnum<visa-resource-name>)  [unwired: 1 in]
  n253 = property class="VISAName"(reference=w211) -> (reference out=w204:refnum<vi>, error out=w212:errorcluster, "Value"=w206:refnum<visa-resource-name>)  [unwired: 1 in]
  n254 = Close Reference(reference=w225, error in (no error)=w226) -> ()  [unwired: 1 out]
  n255 = Close Reference(reference=w224, error in (no error)=w223) -> ()  [unwired: 1 out]
  n256 = Close Reference(reference=w217, error in (no error)=w218) -> ()  [unwired: 1 out]
  n257 = Close Reference(reference=w209, error in (no error)=w216) -> ()  [unwired: 1 out]
  n258 = Close Reference(reference=w205, error in (no error)=w213) -> ()  [unwired: 1 out]
  n259 = Close Reference(reference=w204, error in (no error)=w212) -> ()  [unwired: 1 out]
  n260 = property class="DigNum (strict)"(reference=w178) -> (reference out=w180:refnum<vi>, error out=w179:errorcluster, "Value"=w147:dbl)  [unwired: 1 in]
  n261 = property class="DigNum (strict)"(reference=w177) -> (reference out=w175:refnum<vi>, error out=w176:errorcluster, "Value"=w146:dbl)  [unwired: 1 in]
  n262 = property class="DigNum (strict)"(reference=w172) -> (reference out=w174:refnum<vi>, error out=w173:errorcluster, "Value"=w145:dbl)  [unwired: 1 in]
  n263 = property class="DigNum (strict)"(reference=w171) -> (reference out=w169:refnum<vi>, error out=w170:errorcluster, "Value"=w144:dbl)  [unwired: 1 in]
  n264 = property class="DigNum (strict)"(reference=w167) -> (reference out=w153:refnum<vi>, error out=w168:errorcluster, "Value"=w143:dbl)  [unwired: 1 in]
  n265 = property class="DigNum (strict)"(reference=w166) -> (reference out=w154:refnum<vi>, error out=w165:errorcluster, "Value"=w142:dbl)  [unwired: 1 in]
  n266 = property class="DigNum (strict)"(reference=w163) -> (reference out=w152:refnum<vi>, error out=w164:errorcluster, "Value"=w141:dbl)  [unwired: 1 in]
  n267 = property class="DigNum (strict)"(reference=w162) -> (reference out=w151:refnum<vi>, error out=w161:errorcluster, "Value"=w140:dbl)  [unwired: 1 in]
  n268 = property class="DigNum (strict)"(reference=w159) -> (reference out=w150:refnum<vi>, error out=w160:errorcluster, "Value"=w139:dbl)  [unwired: 1 in]
  n269 = property class="DigNum (strict)"(reference=w157) -> (reference out=w149:refnum<vi>, error out=w158:errorcluster, "Value"=w138:dbl)  [unwired: 1 in]
  n270 = property class="DigNum (strict)"(reference=w156) -> (reference out=w148:refnum<vi>, error out=w155:errorcluster, "Value"=w137:dbl)  [unwired: 1 in]
  n271 = property class="DigNum (strict)"(reference=w14) -> (reference out=w22:refnum<vi>, error out=w15:errorcluster, "Value"=w26:dbl)  [unwired: 1 in]
  n272 = property class="DigNum (strict)"(reference=w17) -> (reference out=w23:refnum<vi>, error out=w16:errorcluster, "Value"=w27:dbl)  [unwired: 1 in]
  n273 = property class="DigNum (strict)"(reference=w19) -> (reference out=w24:refnum<vi>, error out=w18:errorcluster, "Value"=w28:dbl)  [unwired: 1 in]
  n274 = property class="DigNum (strict)"(reference=w20) -> (reference out=w25:refnum<vi>, error out=w21:errorcluster, "Value"=w29:dbl)  [unwired: 1 in]
  n275 = Insert Into Array(array=string[] [], new element #1=w221, new element #2=w220, new element #3=w210, new element #4=w208, new element #5=w207, new element #6=w206) -> (w400:string[])  [unwired: 1 in]
  n276 = for {
    tunnel: w404 -> [w435]
    tunnel: "COM PORT" ("WRITE /READ SECTION") -> [w434]
    tunnel: [w433] -> w181
    tunnel: string[] ["HUMIDITY PORT", "TEMP MODBUS", "HEAVE AND SURGE COM PORT", "SWAY COM PORT", "RAMP PORT", "ECR PORT"] -> [w431] mode=indexing
    tunnel: w400 -> [w430] mode=indexing
    n277 = call "CONFIG FILE MAIN Unitest.vi"("WRITE /READ SECTION"=w434, "WRITE KEY"=w431, "WRITE VALUE"=w430, "error in"=w435, "PARAMETER/CONFIG"=TRUE, "Config Enum"=Config_file__FGV_Unitest_enum."WRITE") -> ("error out"=w433:errorcluster)  [unwired: 12 in, 1 out]
  }
  n278 = Close Reference(reference=w180, error in (no error)=w179) -> ()  [unwired: 1 out]
  n279 = Close Reference(reference=w175, error in (no error)=w176) -> ()  [unwired: 1 out]
  n280 = Close Reference(reference=w174, error in (no error)=w173) -> ()  [unwired: 1 out]
  n281 = Close Reference(reference=w169, error in (no error)=w170) -> ()  [unwired: 1 out]
  n282 = Close Reference(reference=w153, error in (no error)=w168) -> ()  [unwired: 1 out]
  n283 = Close Reference(reference=w154, error in (no error)=w165) -> ()  [unwired: 1 out]
  n284 = Close Reference(reference=w152, error in (no error)=w164) -> ()  [unwired: 1 out]
  n285 = Close Reference(reference=w151, error in (no error)=w161) -> ()  [unwired: 1 out]
  n286 = Close Reference(reference=w150, error in (no error)=w160) -> ()  [unwired: 1 out]
  n287 = Close Reference(reference=w149, error in (no error)=w158) -> ()  [unwired: 1 out]
  n288 = Close Reference(reference=w148, error in (no error)=w155) -> ()  [unwired: 1 out]
  n289 = Close Reference(reference=w22, error in (no error)=w15) -> ()  [unwired: 1 out]
  n290 = Close Reference(reference=w23, error in (no error)=w16) -> ()  [unwired: 1 out]
  n291 = Close Reference(reference=w24, error in (no error)=w18) -> ()  [unwired: 1 out]
  n292 = Close Reference(reference=w25, error in (no error)=w21) -> ()  [unwired: 1 out]
  n293 = Number To Fractional String(number=w147, precision (6)=w13) -> (F-format string=w135:string)  [unwired: 2 in]
  n294 = Number To Fractional String(number=w146, precision (6)=w13) -> (F-format string=w134:string)  [unwired: 2 in]
  n295 = Number To Fractional String(number=w145, precision (6)=w13) -> (F-format string=w133:string)  [unwired: 2 in]
  n296 = Number To Fractional String(number=w144, precision (6)=w13) -> (F-format string=w132:string)  [unwired: 2 in]
  n297 = Number To Fractional String(number=w143, precision (6)=w13) -> (F-format string=w131:string)  [unwired: 2 in]
  n298 = Number To Fractional String(number=w142, precision (6)=w13) -> (F-format string=w130:string)  [unwired: 2 in]
  n299 = Number To Fractional String(number=w141, precision (6)=w13) -> (F-format string=w129:string)  [unwired: 2 in]
  n300 = Number To Fractional String(number=w140, precision (6)=w13) -> (F-format string=w128:string)  [unwired: 2 in]
  n301 = Number To Fractional String(number=w139, precision (6)=w13) -> (F-format string=w127:string)  [unwired: 2 in]
  n302 = Number To Fractional String(number=w138, precision (6)=w13) -> (F-format string=w126:string)  [unwired: 2 in]
  n303 = Number To Fractional String(number=w137, precision (6)=w13) -> (F-format string=w125:string)  [unwired: 2 in]
  n304 = Number To Fractional String(number=w26, precision (6)=w13) -> (F-format string=w12:string)  [unwired: 2 in]
  n305 = Number To Fractional String(number=w27, precision (6)=w13) -> (F-format string=w11:string)  [unwired: 2 in]
  n306 = Number To Fractional String(number=w28, precision (6)=w13) -> (F-format string=w10:string)  [unwired: 2 in]
  n307 = Number To Fractional String(number=w29, precision (6)=w13) -> (F-format string=w9:string)  [unwired: 2 in]
  n308 = Insert Into Array(array=string[] [], new element #1=w135, new element #2=w134, new element #3=w133, new element #4=w132, new element #5=w131, new element #6=w130, new element #7=w129, new element #8=w128, new element #9=w127, new element #10=w126, new element #11=w125, new element #12=w12, new element #13=w11, new element #14=w10, new element #15=w9) -> (w124:string[])  [unwired: 1 in]
  n309 = for {
    tunnel: w181 -> [w442]
    tunnel: "NEW PID PARAMETERS" ("WRITE /READ SECTION") -> [w441]
    tunnel: [w440] -> w182
    tunnel: string[] ["PID DELAY (sec)", "Kp", "Ki", "Kd", "Deaadband", "pct_scale", "Init_step", "i_limit", "Max Step Limit", "Min_pos_limit", "Max_pos_limit", "Fine_tune_zone", "min_deadband_floor", "min_finetune_floor", "dynamic_spindle_noise_scalar", "filter_alpha"] -> [w438] mode=indexing
    tunnel: w124 -> [w436] mode=indexing
    n310 = call "CONFIG FILE MAIN Unitest.vi"("WRITE /READ SECTION"=w441, "WRITE KEY"=w438, "WRITE VALUE"=w436, "error in"=w442, "PARAMETER/CONFIG"=TRUE, "Config Enum"=Config_file__FGV_Unitest_enum."WRITE") -> ("error out"=w440:errorcluster)  [unwired: 12 in, 1 out]
  }
  n311 = call "CONFIG FILE MAIN Unitest.vi"("error in"=w182, "Config Enum"=Config_file__FGV_Unitest_enum."CLOSE") -> ("error out"=→"error out":errorcluster)  [unwired: 16 in, 1 out]
